vi "GetLevels.vi"(6 "calc cache":variant, 11 "waveform":waveform(sgl)) -> (2 "levels":T1, 4 "calc cache out":variant)   [LabVIEW 2017, in "AnalysisHelper.lvlib"]
uses:
  <vilib>/addons/InsightCM/Utilities/Analysis/Shared/AnalysisHelper.lvlib
  <vilib>/addons/InsightCM/Utilities/Analysis/Shared/controls/LevelFeatures.ctl
  <vilib>/addons/InsightCM/Utilities/Analysis/Vibration/VibrationAnalysisFunctions.lvlib
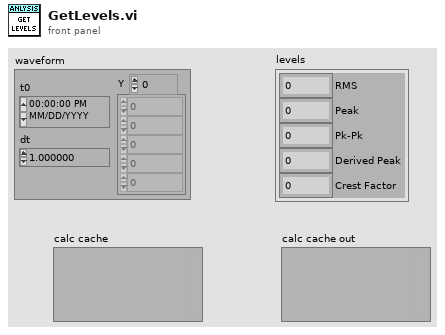
[diagram p1: front panel]
types:
  T1 = typedef "AnalysisHelper.lvlib/LevelFeatures.ctl" = cluster{"RMS":dbl, "Peak":dbl, "Pk-Pk":dbl, "Derived Peak":dbl, "Crest Factor":dbl}
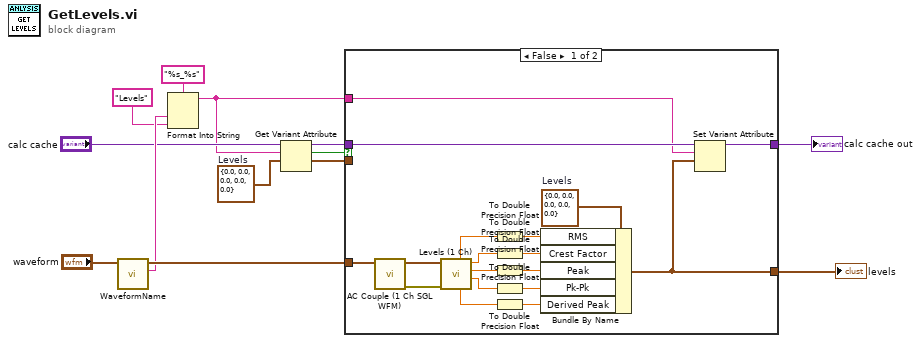
[diagram p0: block diagram]
diagram:
  w12 = T1 {"RMS"=0.0, "Peak"=0.0, "Pk-Pk"=0.0, "Derived Peak"=0.0, "Crest Factor"=0.0}  # Levels
  n1 = call <vilib>:"WaveformName.vi"("signal in"="waveform") -> ("name"=w4:string, "signal out"=w6:waveform(sgl))  [unwired: 9 in]
  n2 = Format Into String(format string="%s_%s", w4, "Levels" ("name")) -> (resulting string=w1:string)  [unwired: 2 in, 1 out]
  n3 = Get Variant Attribute(Variant="calc cache", name=w1, default value (empty Variant)=w12) -> (duplicate Variant=w11:variant, found=w8:bool, value=w9:T1)  [unwired: 1 in, 1 out]
  n4 = case shown="False" w8 {
    tunnel: w6 -> [w31 _]
    tunnel: [w16 w33] -> w13
    tunnel: w11 -> [w17 w32]
    tunnel: w1 -> [w15 _]
    tunnel: [w14 w32] -> w10
    tunnel: w9 -> [_ w33]
    frame False {
      w28 = T1 {"RMS"=0.0, "Peak"=0.0, "Pk-Pk"=0.0, "Derived Peak"=0.0, "Crest Factor"=0.0}  # Levels
      n5 = call <vilib>:"AC Couple (1 Ch SGL WFM).vi"("Signal"=w31) -> ("error out"=w29:errorcluster, "AC Coupled"=w30:waveform(sgl))  [unwired: 8 in, 1 out]
      n6 = call <vilib>:"Levels (1 Ch).vi"("error in (no error)"=w29, "Waveform"=w30) -> ("Pk-Pk"=w21:sgl, "Peak"=w23:sgl, "Crest Factor"=w25:sgl, "Derived Peak"=w19:sgl, "RMS"=w27:sgl)  [unwired: 4 in, 1 out]
      n7 = To Double Precision Float(number=w27) -> (double precision float=w26:dbl)
      n8 = To Double Precision Float(number=w25) -> (double precision float=w24:dbl)
      n9 = To Double Precision Float(number=w23) -> (double precision float=w22:dbl)
      n10 = To Double Precision Float(number=w21) -> (double precision float=w20:dbl)
      n11 = To Double Precision Float(number=w19) -> (double precision float=w18:dbl)
      n12 = Bundle By Name(cluster=w28, "RMS"=w26, "Crest Factor"=w24, "Peak"=w22, "Pk-Pk"=w20, "Derived Peak"=w18) -> (w16:T1)
      n13 = Set Variant Attribute(Variant=w17, name=w15, value=w16) -> (Variant out=w14:variant)  [unwired: 1 in, 2 out]
    }
    frame True {
    }
  }
  "levels" <- w13
  "calc cache out" <- w10
